vi "Open Process Session.vi"(6 "merge output":bool, 7 "stdin":string, 8 "error in (no error)":errorcluster, 9 "working directory":path, 11 "command line":string) -> (0 "error out":errorcluster, 3 "session ID":i32 format="%.0x")   [LabVIEW 2013]
uses:
  ProcessSession.dll
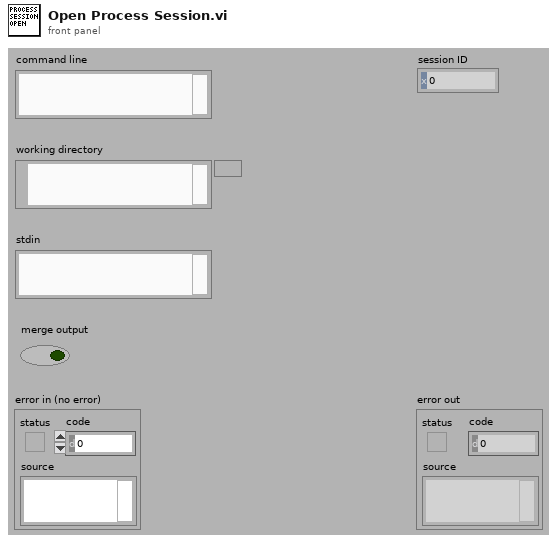
[diagram p1: front panel]
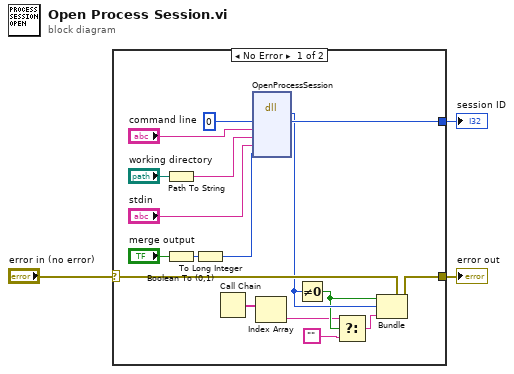
[diagram p0: block diagram]
diagram:
  n1 = case shown="No Error" "error in (no error)" {
    selector: "error in (no error)" -> [w18 w21]
    tunnel: [w19 _] -> w3
    tunnel: [w13 w21] -> w1
    frame No Error {
      n2 = Path To String(path="working directory") -> (string=w8:string)
      n3 = Boolean To (0,1)(Boolean="merge output") -> (0, 1=w5:i16)
      n4 = To Long Integer(number=w5) -> (32bit integer=w4:i32)
      n5 = Call Chain() -> (call chain=w12:string[])
      n6 = dll-call lib="C:/Users/inghoshr/Documents/LabVIEW Data/SmoketestVMVi/Process Session/ProcessSession.dll" fn="OpenProcessSession"("session"=0, "commandLine"="command line", "workingDirectory"=w8, "stdinData"="stdin", "mergeOutput"=w4) -> (w17:i32, "session"=w19:i32)  [unwired: 7 in, 2 out]
      n7 = Index Array(array=w12) -> (element=w11:string)  [unwired: 1 in]
      n8 = Not Equal To 0?(x=w17) -> (x != 0?=w16:bool)
      n9 = Select(t=w11, s=w16, f="") -> (s? t:f=w14:string)
      n10 = Bundle(cluster=w18, "status"=w16, "code"=w17, "source"=w14) -> (w13:errorcluster)
    }
    frame Error {
    }
  }
  "session ID" <- w3
  "error out" <- w1
